vi "EnumInterfacesByGenTL.vi"(0 "error in (no error)":errorcluster caption="错误输入（无错误）", 1 "strGenTLPath":string) -> (2 "error out":errorcluster caption="错误输出", 3 "function return":i32 format="%x", 4 "nInterfaceNum":u32, 5 "pGenTLIfInfoArray":T1(array[cluster]))   [LabVIEW 2013, in "MvCameraControl.lvlib"]
uses:
  MvCameraControl.lvlib
  MvCameraPatch.dll
panel:
  in  "pstDevInfoTemp":T2
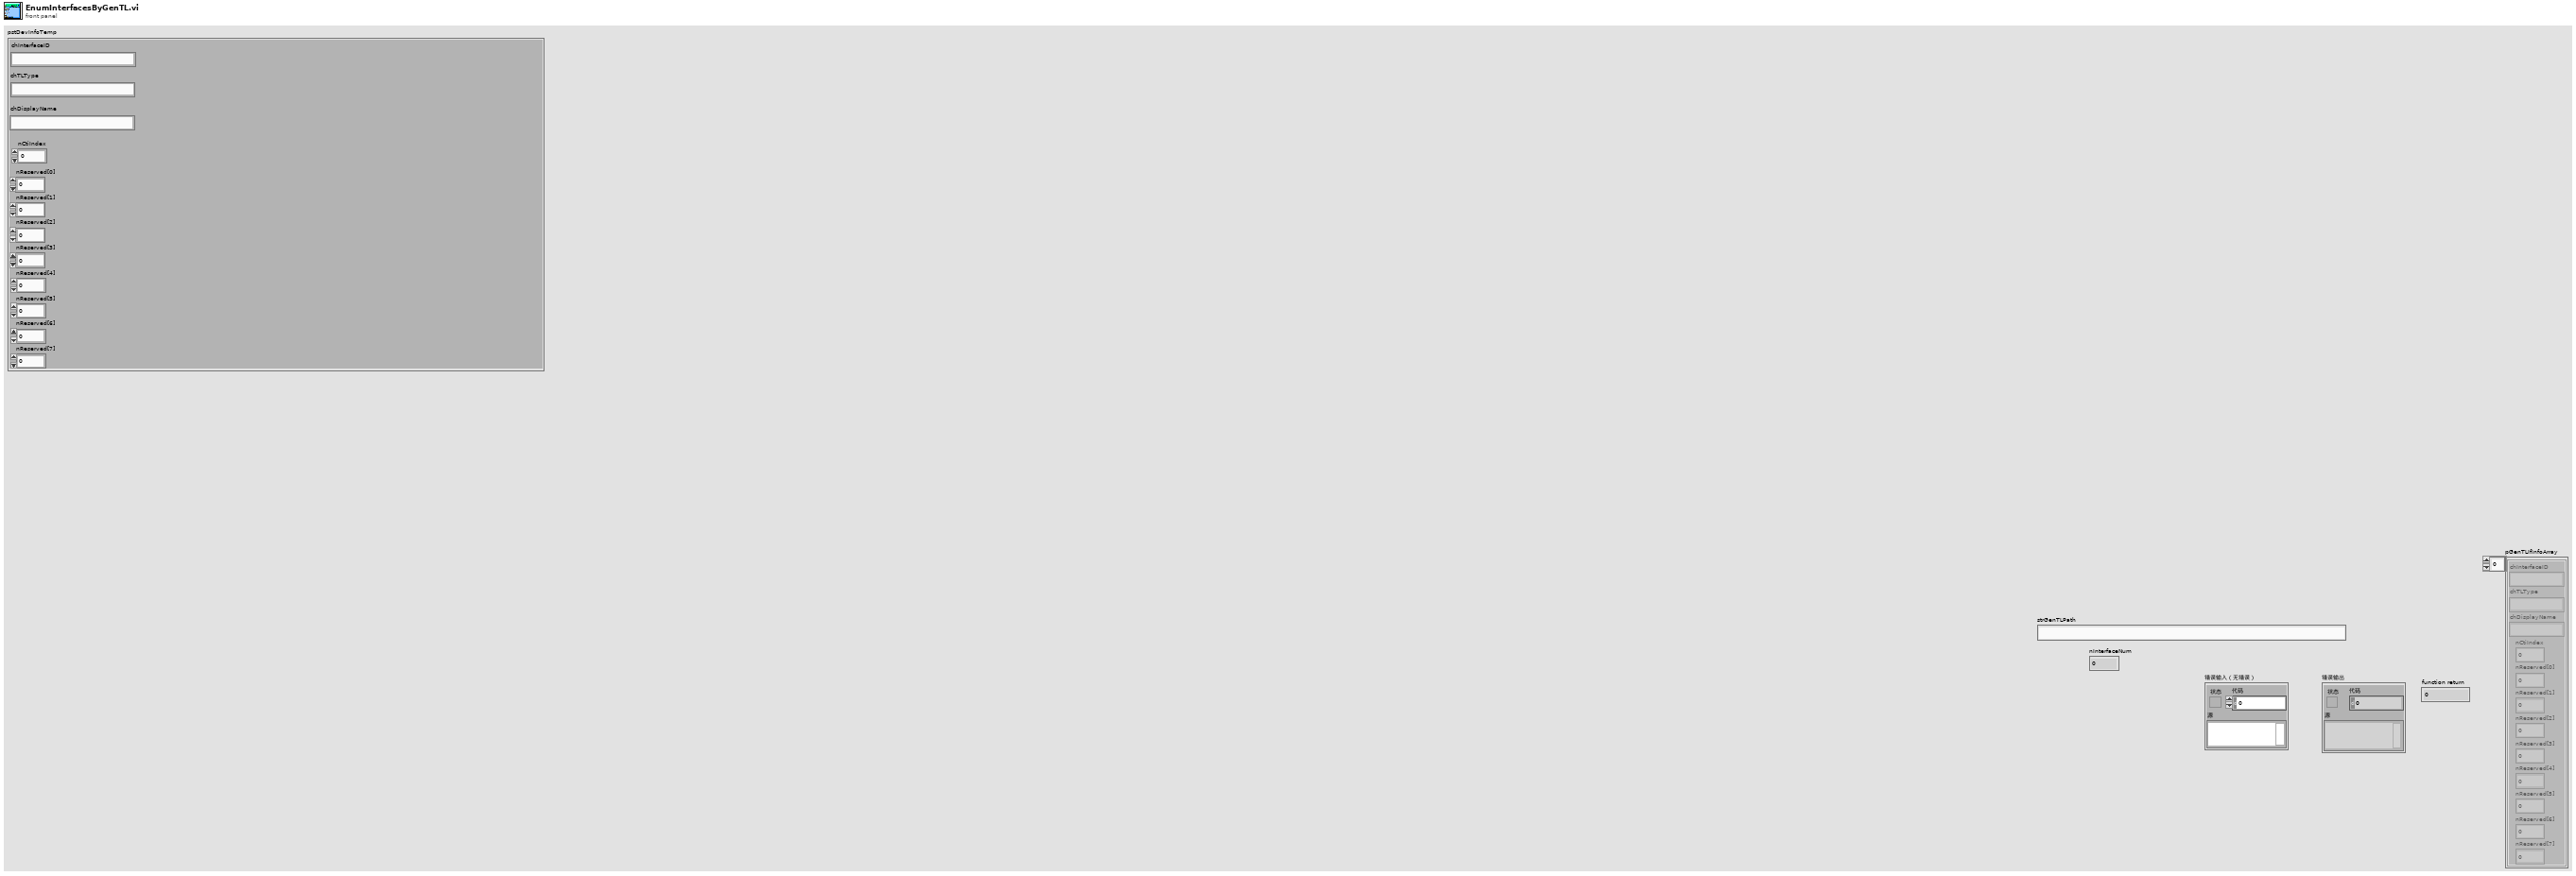
[diagram p1: front panel]
types:
  T1 = cluster{"chInterfaceID":string, "chTLType":string, "chDisplayName":string, "nCtiIndex":u32, "nReserved[0]":u32, "nReserved[1]":u32, "nReserved[2]":u32, "nReserved[3]":u32, "nReserved[4]":u32, "nReserved[5]":u32, "nReserved[6]":u32, "nReserved[7]":u32}[]
  T2 = cluster{"chInterfaceID":string, "chTLType":string, "chDisplayName":string, "nCtiIndex":u32, "nReserved[0]":u32, "nReserved[1]":u32, "nReserved[2]":u32, "nReserved[3]":u32, "nReserved[4]":u32, "nReserved[5]":u32, "nReserved[6]":u32, "nReserved[7]":u32}
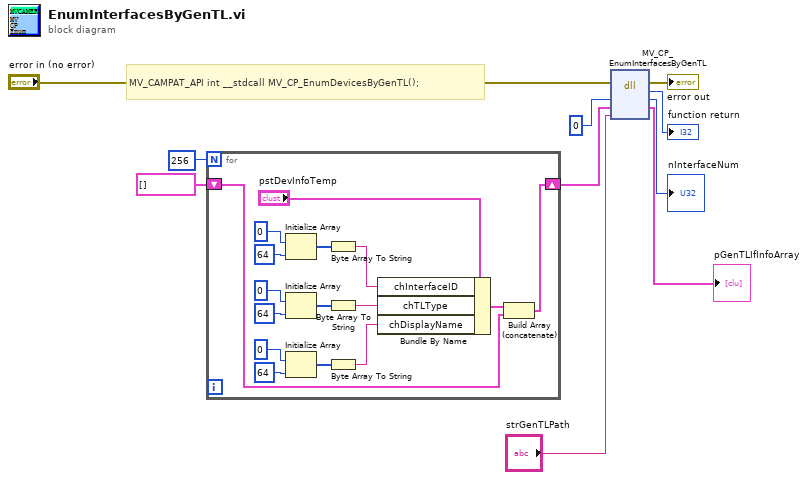
[diagram p0: block diagram]
diagram:
  # "MV_CAMPAT_API int __stdcall MV_CP_EnumDevicesByGenTL();"
  n1 = for {
    N: 256 -> [_]
    shift-right: [w11] -> w8
    shift-left: T1 [] -> [w12]
    n2 = Initialize Array(u8 0 ("元素"), 64 ("维数大小")) -> (w21:u8[])
    n3 = Initialize Array(u8 0 ("元素"), 64 ("维数大小")) -> (w24:u8[])
    n4 = Initialize Array(u8 0 ("元素"), 64 ("维数大小")) -> (w18:u8[])
    n5 = Byte Array To String(unsigned byte array=w21) -> (string=w15:string)
    n6 = Byte Array To String(unsigned byte array=w24) -> (string=w14:string)
    n7 = Byte Array To String(unsigned byte array=w18) -> (string=w13:string)
    n8 = Bundle By Name(cluster="pstDevInfoTemp", "chInterfaceID"=w15, "chTLType"=w14, "chDisplayName"=w13) -> (w17:T2)
    n9 = Build Array (concatenate)(w17, w12) -> (w11:T1)
  }
  n10 = dll-call lib="MvCameraPatch.dll" fn="MV_CP_EnumInterfacesByGenTL"(error in="error in (no error)", "nInterfaceNum"=u32 0, "pGenTLIfInfoArray"=w8, "strGenTLPath"="strGenTLPath") -> (error out=→"error out":errorcluster, "返回类型"=→"function return":i32, "nInterfaceNum"=→"nInterfaceNum":u32, "pGenTLIfInfoArray"=→"pGenTLIfInfoArray":T1)  [unwired: 3 in, 1 out]
